vi "ConvertUnixTimestamp.vi"(11 "Timestamp in":i64) -> (2 "Time Stamp out":timestamp)   [LabVIEW 2017]
doc: "Converts a unix timestamp to a LabVIEW timestamp."
uses:
  <vilib>/Utility/miscctls.llb/LVDateTimeRec.ctl
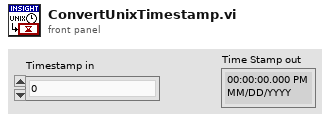
[diagram p1: front panel]
types:
  T1 = typedef "LVDateTimeRec.ctl" = cluster{"fractional second":dbl, "second":i32, "minute":i32, "hour":i32, "day of month":i32, "month":i32, "year":i32, "day of week":i32, "day of year":i32, "DST":i32}
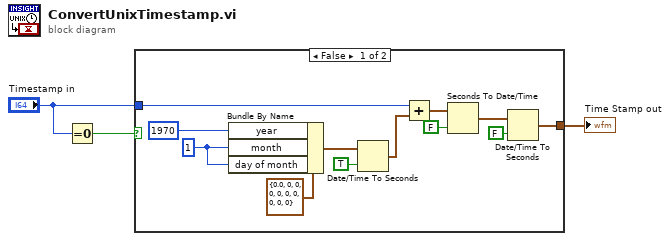
[diagram p0: block diagram]
diagram:
  n1 = Equal To 0?(x="Timestamp in") -> (x = 0?=w3:bool)
  n2 = case shown="False" w3 {
    tunnel: "Timestamp in" -> [w7 _]
    tunnel: [w6 _] -> w1
    frame False {
      w12 = 1 ("month")
      n3 = Bundle By Name(cluster=T1 {"fractional second"=0.0, "second"=0, "minute"=0, "hour"=0, "day of month"=0, "month"=0, "year"=0, "day of week"=0, "day of year"=0, "DST"=0} ("date time rec"), "year"=1970, "month"=w12, "day of month"=w12) -> (w14:T1)
      n4 = Date/Time To Seconds(1:TRUE ("is UTC (F)"), 2:w14) -> (0:w11:timestamp)
      n5 = Add(x=w7, y=w11) -> (x+y=w8:timestamp)
      n6 = Seconds To Date/Time(time stamp (now)=w8, to UTC (F)=FALSE) -> (date time rec=w10:T1)
      n7 = Date/Time To Seconds(1:FALSE ("is UTC (F)"), 2:w10) -> (0:w6:timestamp)
    }
    frame True {
    }
  }
  "Time Stamp out" <- w1
